vi "outputs.vi"() -> ()   [LabVIEW 2019]
panel:
  out "Ready_To_Shoot":bool
  out "Magazine_On":bool
  out "Shooter":dbl
  out "Kicker":dbl
  out "Magazine":dbl
  out "Intake_On":bool
  out "Intake":dbl
  out "Test Solenoid":bool
  out "Field_Oriented":bool
  out "Confirmed_State":bool[](array[boolean])
  out "Boost_Drive_Current_Limit":bool
  out "Wheel_3_Azimuth_Distance (deg)":dbl
  out "Wheel_1_Azimuth_Distance (deg)":dbl
  out "Wheel_2_Azimuth_Distance (deg)":dbl
  out "Wheel_0_Azimuth_Distance (deg)":dbl
  out "Wheel_3_Power":dbl
  out "Wheel_1_Power":dbl
  out "Wheel_2_Power":dbl
  out "Wheel_0_Power":dbl
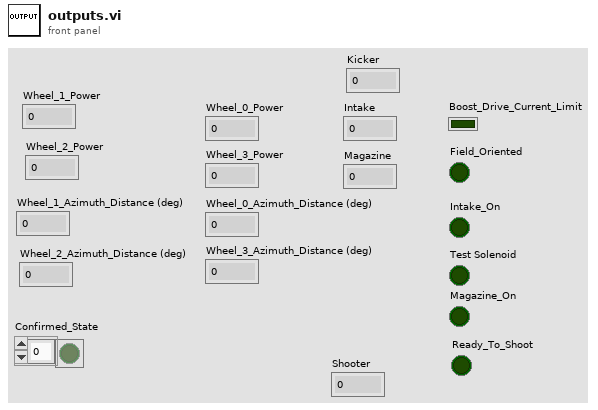
[diagram p1: front panel]
diagram:
